vi "Interface.vi"(8 "error in (no error)":errorcluster, 11 "launcher in":refnum<class "launcher.lvclass">) -> (0 "error out":errorcluster)   [LabVIEW 2021, in "launcher.lvclass"]
uses:
  launcher.lvclass
  C:/Program Files (x86)/National Instruments/LabVIEW 2021/user.lib/S2 Labs/Module Framework/Modules/Base/Module.lvclass
  <userlib>/S2 Labs/CVT Toolkit/CVT.lvclass/CVT.ctl
  MB Slave Simulator Base/TypeDefs/set_register_cmd_type.ctl
  <userlib>/S2 Labs/Queued State Machine/TypeDefs/Queue Message.ctl
  <userlib>/S2 Labs/Queued State Machine/TypeDefs/States.ctl
  <userlib>/S2 Labs/Module Framework/Modules/Base/Module.lvclass/Module.ctl
  <userlib>/S2 Labs/Queued State Machine/QSM.lvclass/QSM.ctl
  <userlib>/S2 Labs/Queued State Machine/Callback Notifier/Callback Notifier.lvclass/Callback Notifier.ctl
  63e6b6d3-4161-417f-9354-0ed5a3a4c731.vi
  b9b6e22c-0ff7-4e2a-8481-ca9931ba087e.vi
  b616af44-0ddf-4500-9638-0b6950c56cf0.vi
  a939f951-0f46-4e98-be35-de35e5f9362a.vi
  d4968b2e-a314-4458-80d5-dad6945f50bf.vi
  63e6b6d3-4161-417f-9354-0ed5a3a4c731.vi/1553f4ce-967c-4f57-a913-5f155bf4374d.vi
  b9b6e22c-0ff7-4e2a-8481-ca9931ba087e.vi/1553f4ce-967c-4f57-a913-5f155bf4374d.vi
  a939f951-0f46-4e98-be35-de35e5f9362a.vi/a5442550-30ab-4f7c-a4e8-4e040bcf3d57.vi
  <userlib>/S2 Labs/Module Framework/Modules/Base/Read Queue.vi
  a939f951-0f46-4e98-be35-de35e5f9362a.vi/77abbf80-a0d7-431e-91bd-d2268efe8bf3.vi
  a939f951-0f46-4e98-be35-de35e5f9362a.vi/7a27d807-84e4-485a-8ba6-289735576614.vi
  <userlib>/S2 Labs/Queued State Machine/Callback Notifier/Read Callback Notifier Ref.vi
  <userlib>/S2 Labs/CVT Toolkit/Read CVT DVR.vi
  <userlib>/S2 Labs/Queued State Machine/Enqueue Element.vi
  Global.vi
  <userlib>/S2 Labs/Module Framework/Modules/Base/Get Module CVT Ref.vi
  <userlib>/S2 Labs/Module Framework/Modules/Base/Get Module Queues Map.vi
  <userlib>/S2 Labs/Queued State Machine/Callback Notifier/Obtain Callback Notifier.vi
  <userlib>/S2 Labs/Queued State Machine/Callback Notifier/Release Reply Notifier.vi
  <vilib>/JDP Science/JSONtext/Variant to JSON Text.vi
  <userlib>/S2 Labs/Alarms and Events Toolkit/Alarms/Set User Event.vi
  <vilib>/Utility/error.llb/Error Cluster From Error Code.vi
  Dialogs/Dialog_EditFormulas.vi
  <userlib>/S2 Labs/Queued State Machine/QSM.lvclass
  <userlib>/S2 Labs/Queued State Machine/Callback Notifier/Callback Notifier.lvclass
  <vilib>/JDP Science/JSONtext/LVClass Serializer/JSONtext LVClass Serializer.lvclass
  <userlib>/S2 Labs/Module Framework/Modules/Base/Module.lvclass
  <userlib>/S2 Labs/CVT Toolkit/CVT.lvclass
  MB Slave Simulator Base/MB Slave Simulator Base.lvclass
panel:
  in  "Tab":enum32{"System Resources", "Data"}(tab)
  out "FPGA User LED":bool
  out "SysResources":T1(graph)
  out "Time Stamp":timestamp
  in  "Edit Formulas":bool
  in  "Set Value":bool
  in  "Value":dbl
  out "Label":string
  in  "System Net Current (A)":dbl(slide) scale=-1000.0..1000.0
  in  "Data Table":i32(listbox) caption="Alarms Table"
  in  "Filter":string
  in  "Module":string(combo)="launcher"
  out "ts":timestamp
  out "Version":string
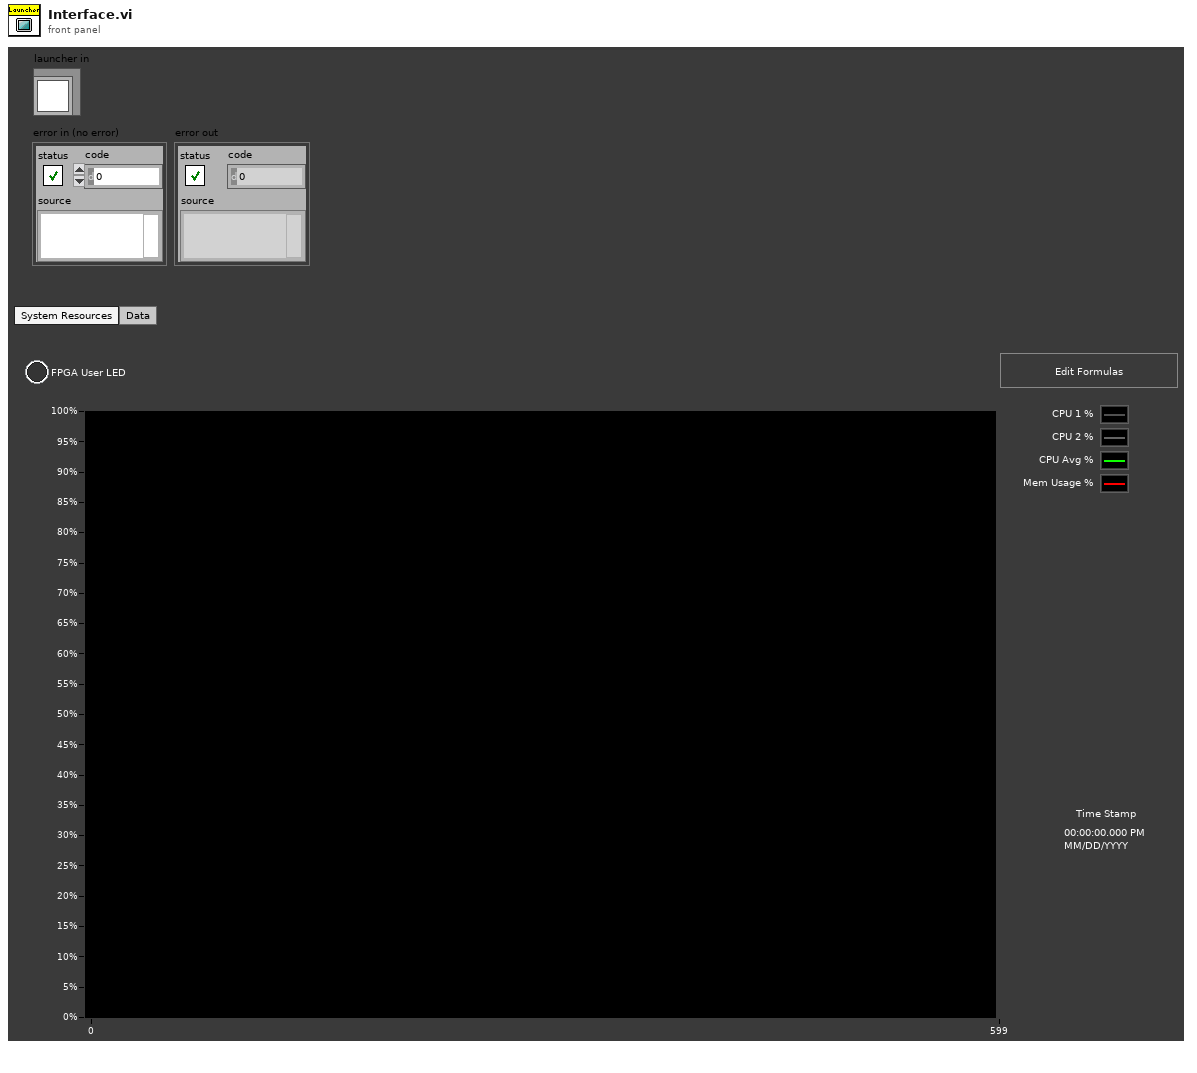
[diagram p1: front panel]
types:
  T1 = cluster{"value":dbl, "value":dbl, "value":dbl, "value":dbl}
  T2 = typedef "QSM.lvclass/Queue Message.ctl" = cluster{"State":T3, "Command":string, "Parameter":variant}
  T3 = typedef "QSM.lvclass/States.ctl" = enum16{"Waiting", "Init", "ExecCMD", "Read Config", "Write Config", "Launch", "Connect", "Recovery", "Clean Up", "Exit"}
  T4 = typedef "MB Slave Simulator Base.lvclass/set_register_cmd_type.ctl" = cluster{"Label":string, "Value":dbl}
  T5 = typedef "CVT.lvclass/Data Cluster.ctl" = cluster{"value":dbl, "ts":timestamp, "variant":variant, "custom value?":bool}
  T6 = cluster{"CVT Name":string, "CVT Data Map":map{string, T5}}[]
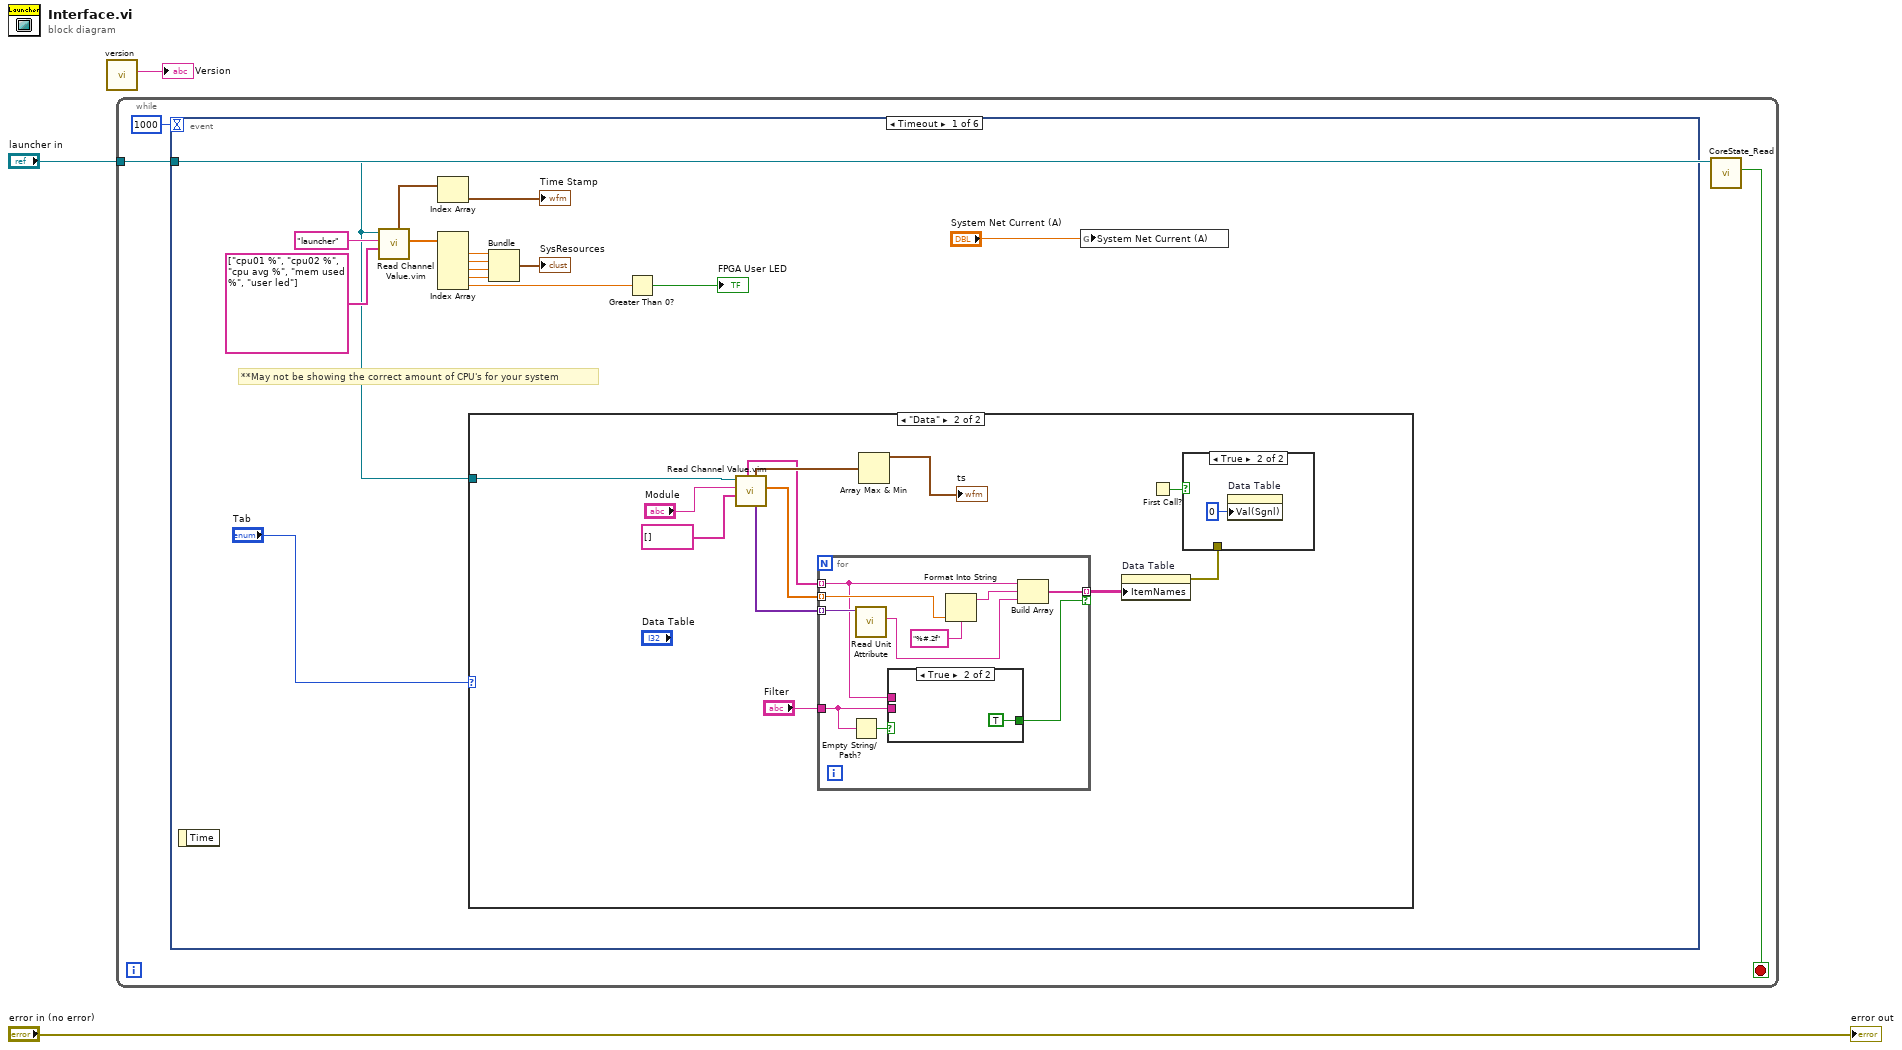
[diagram p0: block diagram]
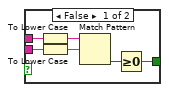
[diagram p4: hidden frame]
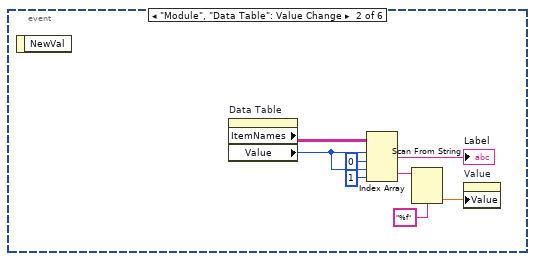
[diagram p5: hidden frame]
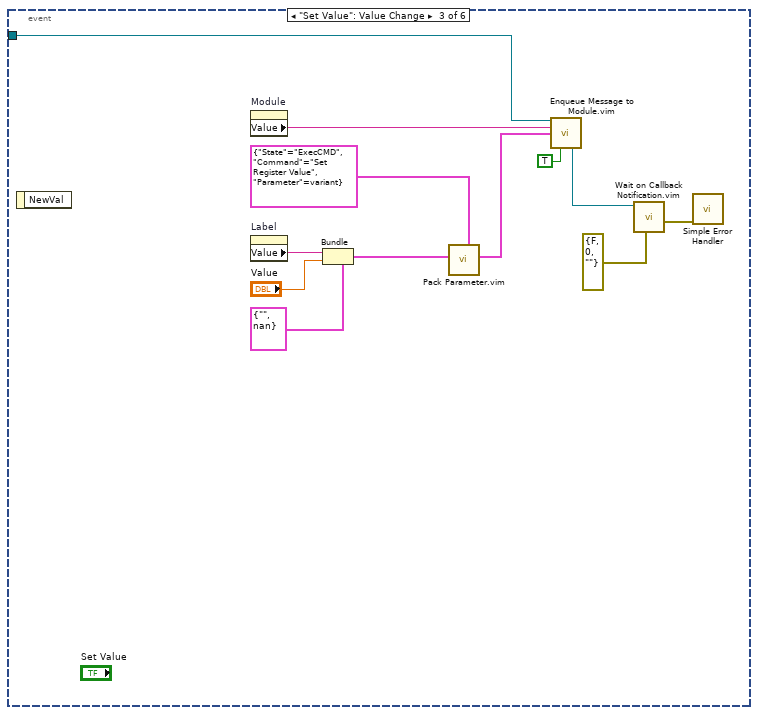
[diagram p6: hidden frame]
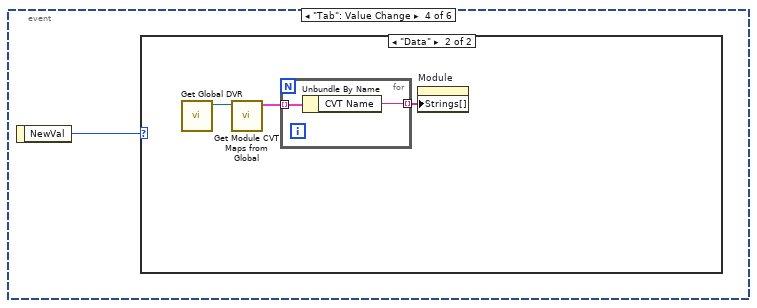
[diagram p7: hidden frame]
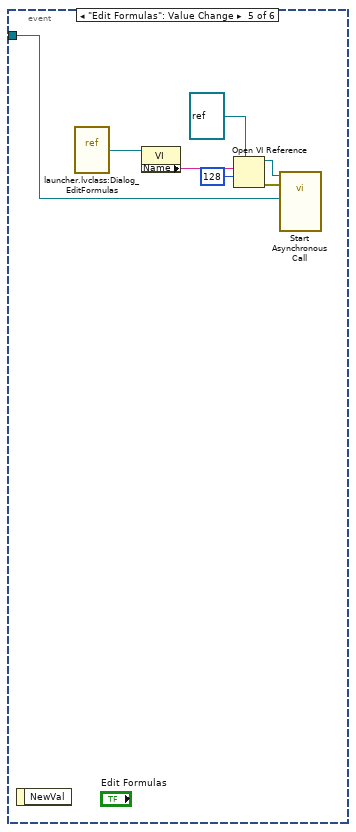
[diagram p9: hidden frame]
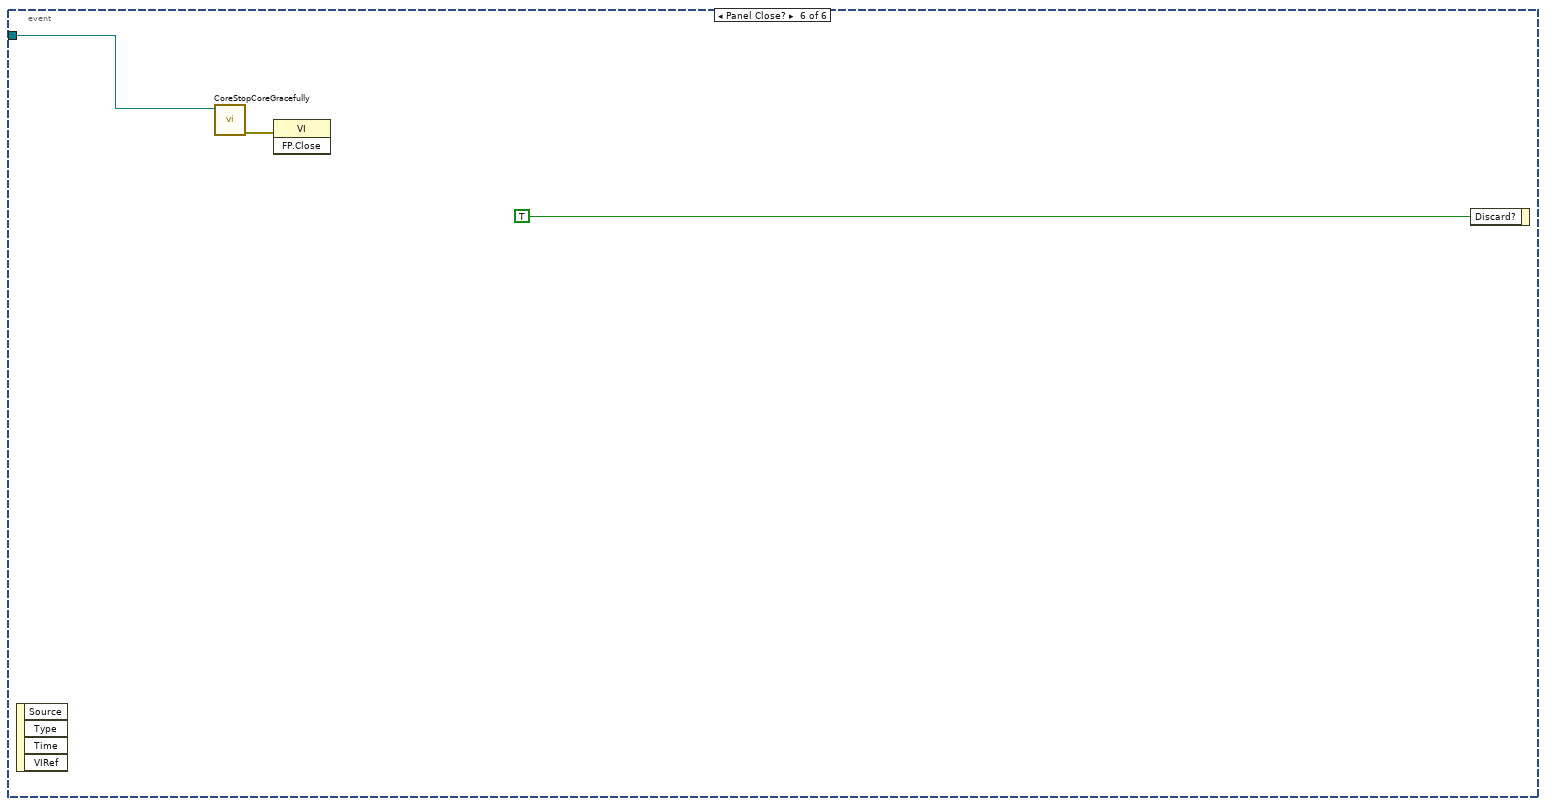
[diagram p10: hidden frame]
diagram:
  n1 = call "version.vi"() -> ("version"=→"Version":string)  [unwired: 11 in]
  n2 = while {
    tunnel: "launcher in" -> [w5]
    stop <- w4 stop-if-true
    n3 = event shown="[0] Timeout" {
      selector: _ -> [_ _ _ _ _ _]
      dyn-events: _ -> [_ _ _ _ _ _]
      timeout: 1000 -> [_ _ _ _ _ _]
      tunnel: w5 -> [w10 _ w71 _ w78 w86]
      event Timeout {
        # "**May not be showing the correct amount of CPU's for your system"
        n4 = event-data() -> ()  [unwired: 1 in, 1 out]
        n5 = call "Read Channel Value.vim"("Channel Label(s)"=string[] ["cpu01 %", "cpu02 %", "cpu avg %", "mem used %", "user led"], "Module"="launcher", "Module in"=w10) -> ("value"=w15:dbl[], "ts"=w14:timestamp[])  [unwired: 2 in, 5 out]
        n6 = Index Array(array=w14) -> (element=→"Time Stamp":timestamp)  [unwired: 1 in]
        n7 = Index Array(array=w15) -> (element #1=w19:dbl, element #2=w18:dbl, element #3=w17:dbl, element #4=w16:dbl, element #5=w8:dbl)  [unwired: 5 in]
        n8 = case shown="\"Data\"" "Tab" {
          tunnel: w10 -> [_ w25]
          frame "System Resources", Default {
          }
          frame "Data" {
            n9 = call "Read Channel Value.vim"("Channel Label(s)"=string[] [], "Module"="Module", "Module in"=w25) -> ("value"=w28:dbl[], "Custom Value"=w29:variant[], "ts"=w31:timestamp[], "Channel Labels*"=w27:string[])  [unwired: 2 in, 3 out]
            n10 = for {
              tunnel: w27 -> [w37] mode=indexing
              tunnel: w28 -> [w42] mode=indexing
              tunnel: w29 -> [w44] mode=indexing
              tunnel: [w39] -> w23 mode=indexing if=w35
              tunnel: "Filter" -> [w36]
              n11 = Empty String/Path?(string/path=w36) -> (empty?=w38:bool)
              n12 = call <userlib>:"Read Unit Attribute.vi"("variant"=w44) -> ("unit"=w40:string)  [unwired: 9 in, 1 out]
              n13 = case shown="True" w38 {
                tunnel: w37 -> [w50 _]
                tunnel: w36 -> [w49 _]
                tunnel: [w47 TRUE] -> w35
                frame False {
                  n14 = To Lower Case(string=w50) -> (all lower case string=w46:string)
                  n15 = To Lower Case(string=w49) -> (all lower case string=w45:string)
                  n16 = Match Pattern(string=w46, regular expression=w45) -> (offset past match=w48:i32)  [unwired: 1 in, 3 out]
                  n17 = Greater Or Equal To 0?(x=w48) -> (x >= 0?=w47:bool)
                }
                frame True {
                }
              }
              n18 = Format Into String(format string="%#.2f", w42) -> (resulting string=w41:string)  [unwired: 2 in, 1 out]
              n19 = Build Array(w37, w41, w40) -> (w39:string[])
            }
            n20 = Array Max & Min(array=w31) -> (max value=→"ts":timestamp)  [unwired: 3 out]
            n21 = property on="Data Table" class="MCListbox (strict)"("ItemNames"=w23) -> (error out=w22:errorcluster)  [unwired: 2 in, 1 out]
            n22 = First Call?() -> (First Call?: T/F=w24:bool)
            n23 = case shown="True" w24 {
              tunnel: w22 -> [_ _]
              frame False {
              }
              frame True {
                n24 = property on="Data Table" class="MCListbox (strict)"("Val(Sgnl)"=0 ("Value (Signaling)")) -> ()  [unwired: 2 in, 2 out]
              }
            }
          }
        }
        n25 = Bundle("value"=w19, "value"=w18, "value"=w17, "value"=w16) -> (→"SysResources":T1)  [unwired: 1 in]
        n26 = Greater Than 0?(x=w8) -> (x > 0?=→"FPGA User LED":bool)
        n27 = global write "Global.vi" "System Net Current (A)"("System Net Current (A)") -> ()
      }
      event "Module", "Data Table": Value Change {
        n28 = event-data() -> ()  [unwired: 1 in, 1 out]
        n29 = property on="Data Table" class="MCListbox (strict)"() -> ("ItemNames"=w59:string[][], "Value"=w57:i32)  [unwired: 2 in, 2 out]
        n30 = Index Array(array=w59, index (row) #1=w57, index (col) #1=0 ("disabled index (col)"), index (row) #2=w57, index (col) #2=1 ("disabled index (col)")) -> (element #1=→"Label":string, element #2=w54:string)
        n31 = Scan From String(format string="%f", input string=w54) -> (output 1=w53:dbl)  [unwired: 3 in, 3 out]
        n32 = property on="Value" class="DigNum (strict)"("Value"=w53) -> ()  [unwired: 2 in, 2 out]
      }
      event "Set Value": Value Change {
        n33 = event-data() -> ()  [unwired: 1 in, 1 out]
        n34 = property on="Module" class="CmbBox"() -> ("Value"=w69:string)  [unwired: 2 in, 2 out]
        n35 = property on="Label" class="Str"() -> ("Value"=w67:string)  [unwired: 2 in, 2 out]
        n36 = Bundle(cluster=T4 {"Label"="", "Value"=nan} ("Set Register CMD"), "Label"=w67, "Value"="Value") -> (w63:T4)
        n37 = call "Pack Parameter.vim"("Message Cluster In"=T2 {"State"=enum."ExecCMD", "Command"="Set Register Value", "Parameter"=variant} ("Message"), "Parameter (string)"=w63) -> ("Message Cluster Out"=w64:T2)  [unwired: 9 in]
        n38 = call "Enqueue Message to Module.vim"("Module in"=w71, "Module Name (self)"=w69, "Message"=w64, "Request Callback Notification? (F)"=TRUE) -> ("Callback Notifier"=w62:refnum<class "Callback Notifier.lvclass">)  [unwired: 6 in, 5 out]
        n39 = call "Wait on Callback Notification.vim"("type (string)"=errorcluster {"status"=FALSE, "code"=0, "source"=""} ("error in (no error)"), "Callback Notifier in"=w62) -> ("notification"=w60:errorcluster)  [unwired: 6 in, 3 out]
        n40 = call <vilib>:"Simple Error Handler.vi"("error in (no error)"=w60) -> ()  [unwired: 4 in, 5 out]
      }
      event "Tab": Value Change {
        n41 = event-data() -> ("NewVal"=w72:enum32{"System Resources", "Data"})  [unwired: 1 in]
        n42 = case shown="\"Data\"" w72 {
          frame "System Resources", Default {
          }
          frame "Data" {
            n43 = call <userlib>:"Get Global DVR.vi"() -> ("Global DVR"=w75:refnum<data-value>)  [unwired: 11 in]
            n44 = call <userlib>:"Get Module CVT Maps from Global.vi"("Global DVR"=w75) -> ("Module CVT Maps"=w74:T6)  [unwired: 9 in, 1 out]
            n45 = for {
              tunnel: w74 -> [w77] mode=indexing
              tunnel: [w76] -> w73 mode=indexing
              n46 = Unbundle By Name(w77) -> ("CVT Name"=w76:string)
            }
            n47 = property on="Module" class="CmbBox"("Strings[]"=w73) -> ()  [unwired: 2 in, 2 out]
          }
        }
      }
      event "Edit Formulas": Value Change {
        n48 = event-data() -> ()  [unwired: 1 in, 1 out]
        n49 = vi-ref "launcher.lvclass:Dialog_EditFormulas.vi"() -> (w80:refnum<vi>)
        n50 = property class="VI"(reference=w80) -> ("Name"=w81:string)  [unwired: 1 in, 2 out]
        n51 = Open VI Reference(type specifier VI Refnum (for type only)=refnum<vi> refnum, vi path=w81, options=128) -> (vi reference=w82:refnum<vi>, error out=w83:errorcluster)  [unwired: 3 in]
        n52 = call-by-ref "Start Asynchronous Call"(reference=w82, error in=w83, "launcher"=w78) -> ()  [unwired: 10 in, 3 out]
      }
      event Panel Close? {
        n53 = event-data() -> ()  [unwired: 1 in, 4 out]
        n54 = call <userlib>:"CoreStopCoreGracefully.vi"("Module in"=w86) -> ("error out"=w85:errorcluster)  [unwired: 9 in, 1 out]
        n55 = invoke class="VI" method="FP.Close"(error in=w85) -> ()  [unwired: 2 in, 3 out]
        n56 = event-data("Discard?"=TRUE) -> ()  [unwired: 1 in, 1 out]
      }
    }
    n57 = call-dynamic "CoreState_Read.vi"("Module in"=w5) -> ("Stopped?"=w4:bool)  [unwired: 8 in, 2 out]
  }
  "error out" <- "error in (no error)"
